vi "lab5.vi"() -> ()   [LabVIEW 2020]
panel:
  out "x or y":bool
  in  "y 2":bool
  in  "x 2":bool
  out "x xnor y":bool
  in  "y 6":bool
  in  "x 7":bool
  out "x xor y":bool
  in  "y 5":bool
  in  "x 6":bool
  out "x nor  y":bool
  in  "y 4":bool
  in  "x 5":bool
  out "x nand y":bool
  in  "y 3":bool
  in  "x 4":bool
  out "not":bool
  in  "x 3":bool
  out "x and y":bool
  in  "y":bool
  in  "x":bool
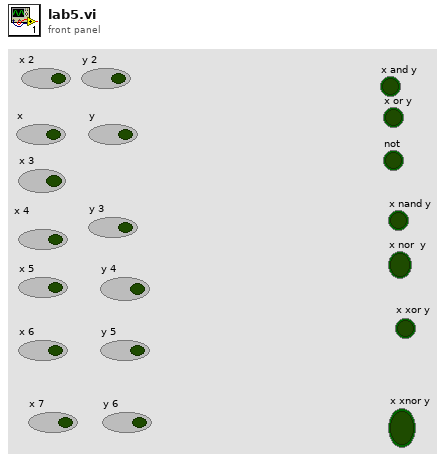
[diagram p1: front panel]
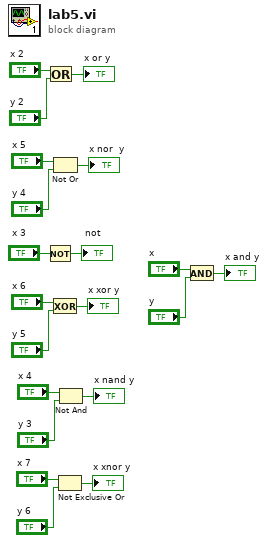
[diagram p0: block diagram]
diagram:
  n1 = Not(x="x 3") -> (.not. x?=→"not":bool)
  n2 = Or(x="x 2", y="y 2") -> (x .or. y?=→"x or y":bool)
  n3 = Not Or(1:"y 4", 2:"x 5") -> (0:→"x nor  y":bool)
  n4 = Exclusive Or(1:"y 5", 2:"x 6") -> (0:→"x xor y":bool)
  n5 = Not Exclusive Or(1:"y 6", 2:"x 7") -> (0:→"x xnor y":bool)
  n6 = Not And(1:"y 3", 2:"x 4") -> (0:→"x nand y":bool)
  n7 = And(x="x", y="y") -> (x .and. y?=→"x and y":bool)
